vi "UHR-Fleezers Control (host) - 12.1.vi"() -> ()   [LabVIEW 2012] (continued)
            n2501 = xnode "Read/Write Control"("FPGA VI Reference In"=w4155, "error in"=w4154, "Green Filter Flipper"=FALSE) -> ("error out"=w4153:errorcluster)  [unwired: 1 out]
          }
        }
      }
      event "Pump 1 contents", "Pump 3 contents": Value Change {
        n2502 = event-data() -> ()  [unwired: 7 out]
        n2503 = local read "Pump 1 contents"() -> (→"Pump 1 cont disp":string)
        n2504 = local read "Pump 3 contents"() -> (→"Pump 3 cont disp":string)
      }
      event "Reset Trap Pos. FB": Value Change {
        n2505 = event-data() -> ()  [unwired: 7 out]
        n2506 = xnode "Read/Write Control"("FPGA VI Reference In"=w4161, "error in"=w4160, "Trap Pos. FB Reset"="Reset Trap Pos. FB") -> ()  [unwired: 2 out]
      }
      event "Rem fb disp offset": Value Change {
        n2507 = event-data() -> ()  [unwired: 7 out]
        n2508 = local write "Rem fb disp offset"(FALSE ("Rem fb disp offset")) -> ()
        n2509 = local read "Mean T1 Position (nm)"() -> (w4163:dbl)
        n2510 = local read "FB Trap Pos Offset"() -> (w4164:dbl)
        n2511 = Subtract(x=w4164, y=w4163) -> (x-y=w4162:dbl)
        n2512 = local write "FB Trap Pos Offset"(w4162) -> ()
      }
      event "Threshold (nm)": Value Change {
        n2513 = event-data() -> ()  [unwired: 7 out]
        n2514 = flat-sequence {
          tunnel: w4168 -> [w4176]
          tunnel: w4167 -> [w4175]
          tunnel: [w4169] -> w4166
          tunnel: w4166 -> [w4182]
          frame #0 {
            n2515 = xnode "Read/Write Control"("FPGA VI Reference In"=w4176, "error in"=w4175) -> ("FPGA VI Reference Out"=w4172:T18, "error out"=w4171:errorcluster, "FPGA TTrig Thresh"=w4173:i64)
            n2516 = local read "Threshold stored (nm)"() -> (w4181:dbl)
            n2517 = local read "Threshold (nm)"() -> (w4169:dbl)
            n2518 = local read "AOM X Cal (nm/MHz)"() -> (w4179:dbl)
            n2519 = Subtract(x=w4169, y=w4181) -> (x-y=w4180:dbl)
            n2520 = Divide(x=w4180, y=w4179) -> (x/y=w4177:dbl)
            n2521 = call "IR AOM freq to word.vi"("Frequency In (MHz)"=w4177) -> ("Frequency Word Out (double)"=w4178:dbl)
            n2522 = To Quad Integer(1:w4178) -> (0:w4174:i64)
            n2523 = Add(x=w4173, y=w4174) -> (x+y=w4170:i64)
            n2524 = xnode "Read/Write Control"("FPGA VI Reference In"=w4172, "error in"=w4171, "FPGA TTrig Thresh"=w4170) -> ()  [unwired: 2 out]
          }
          frame #1 {
            "Threshold stored (nm)" <- w4182
          }
        }
      }
      event "FB Trig Integrate": Value Change {
        n2525 = event-data() -> ()  [unwired: 7 out]
        n2526 = local read "FB Trig Integrate"() -> (w4184:u32)
        n2527 = xnode "Read/Write Control"("FPGA VI Reference In"=w4186, "error in"=w4185, "FB Trig Integrate"=w4184) -> ("error out"=w4183:errorcluster)  [unwired: 1 out]
      }
      event "11": Value Change {
        n2528 = event-data() -> ()  [unwired: 7 out]
        n2529 = local read "11"() -> (w4187:bool)
        n2530 = case shown="True" w4187 {
          frame False {
          }
          frame True {
            n2531 = local read "Messages"() -> (w4189:string)
            n2532 = call "Update messages.vi"("Message to add"="You kicked it up to 11!", "Old message string"=w4189) -> ("New message string"=w4190:string)
            n2533 = call <vilib>:"Beep.vi"() -> ()  [unwired: 12 in]
            n2534 = local write "Messages"(w4190) -> ()
          }
        }
      }
      event "Trap Pos. FB ON": Value Change {
        n2535 = event-data() -> ()  [unwired: 7 out]
        n2536 = xnode "Read/Write Control"("FPGA VI Reference In"=w4193, "error in"=w4192, "Force feedback"="Trap Pos. FB ON") -> ()  [unwired: 2 out]
      }
      event "Remove Action Offset": Value Change {
        n2537 = event-data() -> ()  [unwired: 7 out]
        n2538 = local write "Remove Action Offset"(FALSE ("Remove Action Offset")) -> ()
        n2539 = local read "Trap Pos. FB Mult Factor"() -> (w4198:i64)
        n2540 = local read "Trap Pos FB Action"() -> (w4196:i64)
        n2541 = local read "Trap Pos. FB Offset Factor"() -> (w4194:i64)
        n2542 = Multiply(x=w4198, y=w4196) -> (x*y=w4197:i64)
        n2543 = Add(x=w4197, y=w4194) -> (x+y=w4195:i64)
        n2544 = local write "Trap Pos. FB Offset Factor"(w4195) -> ()
        n2545 = xnode "Read/Write Control"("FPGA VI Reference In"=w4201, "error in"=w4200, "Trap Pos. FB Offset Factor"=w4195) -> ()  [unwired: 2 out]
      }
      event "Remove Unwinding Offset": Value Change {
        n2546 = event-data() -> ()  [unwired: 7 out]
        n2547 = local write "Remove Unwinding Offset"(FALSE ("Remove Action Offset")) -> ()
        n2548 = local read "Trap Pos. FB Mult Factor"() -> (w4213:i64)
        n2549 = local read "Trap Pos FB Action"() -> (w4211:i64)
        n2550 = local read "Trap Pos. FB Offset Factor"() -> (w4210:i64)
        n2551 = Multiply(x=w4213, y=w4211) -> (x*y=w4212:i64)
        n2552 = local read "Trap Pos. FB Mult Factor"() -> (w4209:i64)
        n2553 = Add(x=w4212, y=w4210) -> (x+y=w4203:i64)
        n2554 = Multiply(x=32768, y="factor") -> (x*y=w4206:dbl)
        n2555 = Multiply(x=w4206, y=w4209) -> (x*y=w4208:dbl)
        n2556 = Subtract(x=w4203, y=w4208) -> (x-y=w4207:dbl)
        n2557 = To Quad Integer(1:w4207) -> (0:w4202:i64)
        n2558 = xnode "Read/Write Control"("FPGA VI Reference In"=w4216, "error in"=w4215, "Trap Pos. FB Offset Factor"=w4202) -> ()  [unwired: 2 out]
        n2559 = local write "Trap Pos. FB Offset Factor"(w4202) -> ()
      }
      event "Trap Pos. FB Range", "Trap Pos. FB Gains", "Trap Pos. FB Mult Factor", "Trap Pos. FB Offset Factor", "Trap Pos FB Negate Action", "Trap Pos FB Monitor\nT1 or T2", "Differential FB?", "Negate Diff?": Value Change {
        n2560 = event-data() -> ()  [unwired: 7 out]
        n2561 = Unbundle By Name("Trap Pos. FB Gains") -> ("proportional gain (Kc)"=w4219:fxp<+/-,16,8>, "integral gain (Kc*Ts/Ti)"=w4218:fxp<+/-,16,8>, "derivative gain (Kc*Td/Ts)"=w4217:fxp<+/-,16,8>)
        n2562 = local read "Negate Diff?"() -> (w4224:bool)
        n2563 = Unbundle By Name("Trap Pos. FB Range") -> ("output high"=w4222:fxp<+/-,16,1>, "output low"=w4221:fxp<+/-,16,1>)
        n2564 = xnode "Read/Write Control"("FPGA VI Reference In"=w4232, "error in"=w4231, "FB2 output high"=w4222, "FB2 output low"=w4221, "P2"=w4219, "I2"=w4218, "D2"=w4217, "Trap Pos. FB Mult Factor"="Trap Pos. FB Mult Factor", "Trap Pos. FB Offset Factor"="Trap Pos. FB Offset Factor", "Trap Pos FB Negate Action"="Trap Pos FB Negate Action", "Trap Pos FB Monitor T1 or T2"="Trap Pos FB Monitor\nT1 or T2", "AI1 X Scale"="Trap Pos. AI1 X Pre-scale", "Negate Diff?"=w4224, "Diff FB Measurement?"="Differential FB?") -> ()  [unwired: 2 out]
      }
      event "Trap Pos FB SP", "Trap Pos FB SP 2", "Use SP 2": Value Change {
        n2565 = event-data() -> ()  [unwired: 7 out]
        n2566 = Select(t="Trap Pos FB SP 2", s="Use SP 2", f="Trap Pos FB SP") -> (s? t:f=w4233:fxp<+/-,16,1>)
        n2567 = xnode "Read/Write Control"("FPGA VI Reference In"=w4238, "error in"=w4237, "Trap Pos. FB SP"=w4233) -> ()  [unwired: 2 out]
      }
      event "Offset SP2 from SP1": Value Change {
        n2568 = event-data() -> ()  [unwired: 7 out]
        n2569 = local read "Trap Pos FB SP"() -> (w4241:fxp<+/-,16,1>)
        n2570 = Add(x=w4241, y="SP2 Offset") -> (x+y=w4239:fxp<+/-,16,1>)
        n2571 = property on="Trap Pos FB SP 2" class="DigNum (strict)"("Val(Sgnl)"=w4239) -> ()  [unwired: 2 in, 2 out]
        n2572 = local write "Offset SP2 from SP1"(FALSE ("Offset SP2 from SP1")) -> ()
      }
      event "Set Reading to\nSetpoint": Value Change {
        # "This is the actual PID input signal"
        n2573 = event-data() -> ()  [unwired: 7 out]
        n2574 = local write "Set Reading to\nSetpoint"(FALSE ("Set SP to Reading")) -> ()
        n2575 = xnode "Read/Write Control"("FPGA VI Reference In"=w4247, "error in"=w4246) -> ("FPGA VI Reference Out"=w4245:T18, "error out"=w4244:errorcluster, "Trap Pos FB Int-Norm Signal"=w4243:fxp<+/-,16,1>)
        n2576 = local read "Differential FB?"() -> (w4248:bool)
        n2577 = case shown="False" w4248 {
          tunnel: [w4253 w4260] -> w4250
          tunnel: w4243 -> [w4251 w4260]
          frame False {
            n2578 = local read "Trap Pos FB Monitor\nT1 or T2"() -> (w4256:bool)
            n2579 = local read "Trap X AI1 (DMA)"() -> (w4259:T13)
            n2580 = Unbundle By Name(w4259) -> ("Set 1"=w4258:fxp<+/-,16,1>, "Set 2"=w4257:fxp<+/-,16,1>)
            n2581 = Select(t=w4258, s=w4256, f=w4257) -> (s? t:f=w4255:fxp<+/-,16,1>)
            n2582 = Not(x="Set SP Using...") -> (.not. x?=w4252:bool)
            n2583 = Select(t=w4251, s=w4252, f=w4255) -> (s? t:f=w4253:fxp<+/-,16,1>)
          }
          frame True {
          }
        }
        n2584 = xnode "Read/Write Control"("FPGA VI Reference In"=w4245, "error in"=w4244, "Trap Pos. FB SP"=w4250) -> ()  [unwired: 2 out]
        n2585 = local write "Trap Pos FB SP"(w4250) -> ()
      }
      event "Trap Pos. FB Out Scale 2^n": Value Change {
        n2586 = event-data() -> ()  [unwired: 7 out]
        n2587 = Scale By Power Of 2(n="Trap Pos. FB Out Scale 2^n", x=ext 1.0) -> (x*2^n=w4261:ext)
        n2588 = property on="Trap Pos. FB Mult Factor" class="DigNum (strict)"("Val(Sgnl)"=w4261) -> ()  [unwired: 2 in, 2 out]
      }
      event "Trap Pos FB Int Count": Value Change {
        n2589 = event-data() -> ()  [unwired: 7 out]
        n2590 = xnode "Read/Write Control"("FPGA VI Reference In"=w4266, "error in"=w4265, "Trap Pos FB Int Count"="Trap Pos FB Int Count") -> ()  [unwired: 2 out]
      }
      event "Trap pos": Value Change {
        n2591 = event-data() -> ()  [unwired: 7 out]
        n2592 = case shown="True" "Trap pos" {
          frame False {
            n2593 = property on="Trap Delta Graph" class="WFGraph (strict)"("Visible"=TRUE) -> ()  [unwired: 2 in, 2 out]
            n2594 = property on="Saved trap pos" class="WFGraph (strict)"("Visible"=FALSE) -> ()  [unwired: 2 in, 2 out]
          }
          frame True {
            n2595 = property on="Saved trap pos" class="WFGraph (strict)"("Visible"=TRUE) -> ()  [unwired: 2 in, 2 out]
            n2596 = property on="Trap Delta Graph" class="WFGraph (strict)"("Visible"=FALSE) -> ()  [unwired: 2 in, 2 out]
          }
        }
      }
    }
    "error out 2" <- w3161
    n2597 = node-c288() -> ()  [unwired: 2 out]
  }
  n2598 = timed-loop "Oscillate Trap/AOM (fishing, debugging)" {
    tunnel: w28 -> [w4273]
    tunnel: [w4272] -> w119
    timing: w114 -> [_]
    timing-out: [_] -> w113
    stop <- w4272 stop-if-true
    n2599 = node-c288() -> ()  [unwired: 2 out]
    n2600 = event shown="[0] \"Oscillate Set 1\", \"Fish for Tether\": Value Change" {
      selector: _ -> [_ _ _]
      dyn-events: _ -> [_ _ _]
      timeout: _ -> [_ _ _]
      tunnel: w4273 -> [w4280 _ _]
      tunnel: [FALSE ("Stop All") _ w4869] -> w4272
      event "Oscillate Set 1", "Fish for Tether": Value Change {
        n2601 = event-data() -> ()  [unwired: 6 out]
        n2602 = local read "Oscillate Set 1"() -> (w4279:bool)
        n2603 = Or(x=w4279, y="Fish for Tether") -> (x .or. y?=w4277:bool)
        n2604 = case shown="True" w4277 {
          tunnel: w4280 -> [_ w4283]
          tunnel: "Fish for Tether" -> [_ w4282]
          frame False {
          }
          frame True {
            n2605 = case shown="True" w4282 {
              selector: w4282 -> [w4286 w4292]
              tunnel: [w4286 w4292] -> w4281
              frame False {
              }
              frame True {
                n2606 = local write "Scan axis 2"(TRUE) -> ()
                n2607 = local write "Tether"(FALSE ("Tether")) -> ()
                n2608 = local read "Flow ON during cal?"() -> (w4287:bool)
                n2609 = property on="Trap Delta (MHz)" class="DigNum (strict)"("Val(Sgnl)"="Furthest Delta (MHz)") -> ()  [unwired: 2 in, 2 out]
                n2610 = Or(x="Flow ON during \nfishing?", y=w4287) -> (x .or. y?=w4288:bool)
                n2611 = Wait (ms)(milliseconds to wait=u32 500) -> ()  [unwired: 1 out]
                n2612 = property on="Sample Channel\nFlow" class="Bool (strict)"("Val(Sgnl)"=w4288) -> ()  [unwired: 2 in, 2 out]
              }
            }
            n2613 = node-c288() -> (w4285:T20)  [unwired: 4 out]
            n2614 = timed-loop "Oscillate AOD" {
              timing: w4285 -> [_]
              timing-out: [_] -> w4284
              tunnel: w4283 -> [w4302]
              tunnel: w4281 -> [w4295]
              i -> [w4304]
              stop <- w4301 stop-if-true
              n2615 = node-c288() -> (w4303:i64)  [unwired: 1 out]
              n2616 = flat-sequence {
                tunnel: w4304 -> [w4331]
                tunnel: w4303 -> [w4330]
                tunnel: w4302 -> [w4309]
                tunnel: w4295 -> [w4312]
                tunnel: [w4312] -> w4300
                tunnel: [w4311] -> w4299
                tunnel: [w4308] -> w4298
                tunnel: [w4305] -> w4296
                tunnel: w4300 -> [w4367]
                tunnel: w4299 -> [w4365]
                tunnel: w4298 -> [w4364]
                tunnel: [w4363] -> w4297
                tunnel: w4296 -> [w4362]
                tunnel: [w4439] -> w4301
                tunnel: w4297 -> [w4438]
                frame #0 {
                  n2617 = Divide(x=w4330, y=i64 1000) -> (x/y=w4325:dbl)
                  n2618 = Multiply(x=w4325, y=w4331) -> (x*y=w4327:dbl)
                  n2619 = local read "BD 1 Frequency 2 (MHz)"() -> (w4310:dbl)
                  n2620 = Multiply(x="Osc. freq. (Hz)", y=6.283185307179586) -> (x*y=w4328:dbl)
                  n2621 = Multiply(x=w4328, y=w4327) -> (x*y=w4307:dbl)
                  n2622 = local read "BD 1 Frequency 1 (MHz)"() -> (w4315:dbl)
                  n2623 = local read "BD 2 Frequency 1 (MHz)"() -> (w4314:dbl)
                  n2624 = case shown="True" w4312 {
                    tunnel: w4307 -> [w4337 w4342]
                    tunnel: w4315 -> [_ w4353]
                    tunnel: w4310 -> [_ w4354]
                    tunnel: [w4334 w4348] -> w4313
                    tunnel: [FALSE w4345] -> w4308
                    tunnel: [0.0 w4338] -> w4305
                    frame False {
                      n2625 = Sine(x=w4337) -> (sin(x)=w4335:dbl)
                      n2626 = Multiply(x=w4335, y="Osc. amp. (MHz)") -> (x*y=w4334:dbl)
                    }
                    frame True {
                      n2627 = Cosine(x=w4342) -> (cos(x)=w4357:dbl)
                      n2628 = Subtract(x=w4354, y=w4353) -> (x-y=w4352:dbl)
                      n2629 = Decrement(x=w4357) -> (x-1=w4356:dbl)
                      n2630 = Subtract(x=w4352, y="Closest Delta (MHz)") -> (x-y=w4349:dbl)
                      n2631 = Divide(x=w4356, y=-2.0) -> (x/y=w4350:dbl)
                      n2632 = Multiply(x=w4350, y=w4349) -> (x*y=w4348:dbl)
                      n2633 = local read "Vec Mean of T1 T2"() -> (w4344:dbl[])
                      n2634 = Greater?(x=w4344, y="Stop F (pN)") -> (0:w4346:bool[])
                      n2635 = Or Array Elements(Boolean array=w4346) -> (logical OR=w4345:bool)
                      n2636 = Divide(x=w4342, y=6.283185307179586) -> (x/y=w4341:dbl)
                      n2637 = Round Toward +Infinity(x=w4341) -> (ceil(x): smallest int >= x=w4338:dbl)
                      "Attempts" <- w4338
                      n2638 = Greater?(x=w4338, y="Attempt Limit") -> (0:w4340:bool)
                      n2639 = case shown="True" w4340 {
                        frame False {
                        }
                        frame True {
                          n2640 = local write "Fish for Tether"(FALSE ("Fish for Tether")) -> ()
                          n2641 = call <vilib>:"Beep.vi"() -> ()  [unwired: 3 in, 9 out]
                          n2642 = local read "Messages"() -> (w4359:string)
                          n2643 = call "Update messages.vi"("Message to add"="Tether fishing timeout." ("Messages"), "Old message string"=w4359) -> ("New message string"=→"Messages":string)
                        }
                      }
                    }
                  }
                  n2644 = Select(t=w4315, s="Scan axis 2", f=w4314) -> (s? t:f=w4318:dbl)
                  n2645 = Add(x=w4313, y=w4318) -> (x+y=w4311:dbl)
                  n2646 = Select(t=w4311, s="Scan axis 2", f=w4315) -> (s? t:f=w4321:dbl)
                  n2647 = Select(t=w4314, s="Scan axis 2", f=w4311) -> (s? t:f=w4320:dbl)
                  n2648 = local read "Y RF Frequency Limits (MHz)"() -> (w4316:T15)
                  n2649 = local read "X RF Frequency Limits (MHz)"() -> (w4317:T15)
                  n2650 = local read "BD 1 Frequency 3 (MHz)"() -> (w4324:dbl)
                  n2651 = local read "BD 2 Frequency 2 (MHz)"() -> (w4323:dbl)
                  n2652 = local read "BD 2 Frequency 3 (MHz)"() -> (w4322:dbl)
                  n2653 = call "set RF board frequency - interlace.vi"("Board 2 Frequency Limits"=w4316, "Board 1 Frequency Limits"=w4317, "FPGA VI Reference In"=w4309, "Board 2 Frequency 3 (MHz)"=w4322, "Board 1 Frequency 3 (MHz)"=w4324, "Board 2 Frequency 2 (MHz)"=w4323, "Board 2 Frequency 1 (MHz)"=w4320, "Board 1 Frequency 2 (MHz)"=w4310, "Board 1 Frequency 1  (MHz)"=w4321) -> ()  [unwired: 1 in, 2 out]
                }
                frame #1 {
                  n2654 = And(x=w4367, y=w4364) -> (x .and. y?=w4366:bool)
                  n2655 = case "Only if were fishing and now formed tether" shown="False" w4366 {
                    tunnel: w4365 -> [w4369 w4384]
                    tunnel: [w4368 w4383] -> w4363
                    tunnel: w4362 -> [_ w4379]
                    frame False {
                      n2656 = local read "Fish for Tether"() -> (w4368:bool)
                      n2657 = case shown="False" w4368 {
                        tunnel: w4369 -> [w4370 _]
                        frame False {
                          n2658 = property on="BD 1 Frequency 1 (MHz)" class="DigNum (strict)"("Val(Sgnl)"=w4370) -> ()  [unwired: 2 in, 2 out]
                        }
                        frame True {
                        }
                      }
                    }
                    frame True {
                      w4383 = FALSE ("Fish for Tether")
                      n2659 = call <vilib>:"Beep.vi"() -> ()  [unwired: 3 in, 9 out]
                      n2660 = Number To Decimal String(number=w4379, width (-)=i16 1) -> (decimal integer string=w4377:string)
                      n2661 = Concatenate Strings("Formed tether in ", w4377, " attempt(s)." ("string")) -> (w4374:string)
                      n2662 = local read "Messages"() -> (w4381:string)
                      n2663 = local write "Fish for Tether"(w4383) -> ()
                      n2664 = call "Update messages.vi"("Message to add"=w4374, "Old message string"=w4381) -> ("New message string"=w4380:string)
                      n2665 = local write "Messages"(w4380) -> ()
                      n2666 = Get Date/Time In Seconds() -> (seconds since 1Jan1904=→"Time tether formed":timestamp)
                      n2667 = local read "Flow ON during cal?"() -> (w4371:bool)
                      n2668 = property on="Sample Channel\nFlow" class="Bool (strict)"("Val(Sgnl)"=w4371) -> (error out=w4372:errorcluster)  [unwired: 2 in, 1 out]
                      n2669 = case shown="\"2\", \"3\", \"4\", \"5\", \"6\"" "Then..." {
                        selector: "Then..." -> [_ w4387]
                        tunnel: w4384 -> [w4386 _]
                        tunnel: w4372 -> [_ _]
                        frame "1", Default {
                          n2670 = property on="BD 1 Frequency 1 (MHz)" class="DigNum (strict)"("Val(Sgnl)"=w4386) -> ()  [unwired: 2 in, 2 out]
                        }
                        frame "2", "3", "4", "5", "6" {
                          n2671 = flat-sequence {
                            tunnel: w4387 -> [w4389]
                            frame #0 {
                              n2672 = property on="Trap Delta (MHz)" class="DigNum (strict)"("Val(Sgnl)"="Move to Delta 1 (MHz)") -> ()  [unwired: 2 in, 2 out]
                            }
                            frame #1 {
                              n2673 = case shown="\"5\", \"6\"" w4389 {
                                selector: w4389 -> [w4392 w4402 _]
                                frame "3", "4" {
                                n2674 = flat-sequence {
                                tunnel: w4392 -> [w4393]
                                tunnel: [w4393] -> w4390
                                tunnel: [w4395] -> w4391
                                tunnel: w4390 -> [w4395]
                                tunnel: w4391 -> [w4399]
                                frame #0 {
                                n2675 = property on="Green Laser ON/Interlacing" class="Bool (strict)"("Val(Sgnl)"=TRUE ("Value (Signaling)")) -> ()  [unwired: 2 in, 2 out]
                                }
                                frame #1 {
                                n2676 = Multiply(x="Wait Before Save (s)", y=u32 1000 ("x")) -> (x*y=w4397:u32)
                                n2677 = Wait (ms)(milliseconds to wait=w4397) -> ()  [unwired: 1 out]
                                }
                                frame #2 {
                                n2678 = property on="Start Saving" class="Bool (strict)"("Value"=TRUE ("Start Saving")) -> ()  [unwired: 2 in, 2 out]
                                n2679 = case shown="\"4\"" w4399 {
                                frame Default {
                                }
                                frame "4" {
                                n2680 = property on="Fl. Triggered..." class="Bool (strict)"("Val(Sgnl)"=TRUE ("Value (Signaling)")) -> ()  [unwired: 2 in, 2 out]
                                }
                                }
                                }
                                }
                                }
                                frame "5", "6" {
                                n2681 = stacked-sequence {
                                tunnel: w4402 -> [_ _ _ _ _ _ w4414]
                                frame #0 {
                                n2682 = Replace Array Subset(array=u32[] [0] ("Index Values"), new element="Raster Set Upon Tether", index=0) -> (w4403:u32[])
                                n2683 = property on="Saved AOD Raster Scan Parameter Sets" class="Arr (strict)"("Index Values"=w4403) -> ()  [unwired: 2 in, 2 out]
                                }
                                frame #1 {
                                n2684 = Wait (ms)(milliseconds to wait=u32 500) -> ()  [unwired: 1 out]
                                }
                                frame #2 {
                                n2685 = property on="Load parameters" class="Bool (strict)"("Val(Sgnl)"=TRUE ("Value (Signaling)")) -> ()  [unwired: 2 in, 2 out]
                                n2686 = case shown="True" "Green ON During Raster" {
                                frame False {
                                }
                                frame True {
                                n2687 = property on="Green Laser ON/Interlacing" class="Bool (strict)"("Val(Sgnl)"=TRUE ("Value (Signaling)")) -> ()  [unwired: 2 in, 2 out]
                                }
                                }
                                }
                                frame #3 {
                                n2688 = Wait (ms)(milliseconds to wait=u32 500) -> ()  [unwired: 1 out]
                                }
                                frame #4 {
                                n2689 = property on="Trap Raster Scan" class="Bool (strict)"("Val(Sgnl)"=TRUE ("Value (Signaling)")) -> ()  [unwired: 2 in, 2 out]
                                }
                                frame #5 {
                                n2690 = Wait (ms)(milliseconds to wait=u32 2000) -> ()  [unwired: 1 out]
                                }
                                frame #6 {
                                n2691 = flat-sequence {
                                tunnel: w4414 -> [w4421]
                                frame #0 {
                                n2692 = while {
                                stop <- w4417 stop-if-true
                                n2693 = local read "Raster Scanning..."() -> (w4416:bool)
                                n2694 = local read "Saving..."() -> (w4419:bool)
                                n2695 = Wait (ms)(milliseconds to wait=u32 100) -> ()  [unwired: 1 out]
                                n2696 = Not(x=w4419) -> (.not. x?=w4418:bool)
                                n2697 = Not(x=w4416) -> (.not. x?=w4415:bool)
                                n2698 = And(x=w4418, y=w4415) -> (x .and. y?=w4417:bool)
                                }
                                }
                                frame #1 {
                                n2699 = local read "Tether"() -> (w4422:bool)
                                n2700 = case shown="True" w4422 {
                                tunnel: w4421 -> [_ w4424]
                                frame False {
                                n2701 = property on="Fish for Tether" class="Bool (strict)"("Val(Sgnl)"="Fish again after \nraster break?") -> ()  [unwired: 2 in, 2 out]
                                }
                                frame True {
                                n2702 = stacked-sequence {
                                tunnel: w4424 -> [_ w4428 _ _]
                                frame #0 {
                                n2703 = property on="Trap Delta (MHz)" class="DigNum (strict)"("Val(Sgnl)"="Move to Delta 2 (MHz)") -> ()  [unwired: 2 in, 2 out]
                                n2704 = case shown="True" "Flow ON after\ntether testing?" {
                                frame False {
                                }
                                frame True {
                                n2705 = property on="Sample Channel\nFlow" class="Bool (strict)"("Val(Sgnl)"=TRUE ("Value (Signaling)")) -> ()  [unwired: 2 in, 2 out]
                                }
                                }
                                }
                                frame #1 {
                                n2706 = flat-sequence {
                                tunnel: w4428 -> [w4430]
                                frame #0 {
                                n2707 = Wait (ms)(milliseconds to wait=u32 500) -> ()  [unwired: 1 out]
                                }
                                frame #1 {
                                n2708 = case shown="\"6\"" w4430 {
                                frame Default {
                                }
                                frame "6" {
                                n2709 = property on="Green Laser ON/Interlacing" class="Bool (strict)"("Val(Sgnl)"=TRUE ("Green Laser ON/Interlacing")) -> ()  [unwired: 2 in, 2 out]
                                }
                                }
                                }
                                frame #2 {
                                n2710 = Wait (ms)(milliseconds to wait=u32 500) -> ()  [unwired: 1 out]
                                }
                                frame #3 {
                                n2711 = local write "Start Saving"("Save at end (5, 6)") -> ()
                                }
                                }
                                }
                                frame #2 {
                                n2712 = local read "Bead Sep. Int. Time (s)"() -> (w4436:dbl)
                                n2713 = Multiply(x=w4436, y=1000.0) -> (x*y=w4435:dbl)
                                n2714 = Wait (ms)(milliseconds to wait=w4435) -> ()  [unwired: 1 out]
                                }
                                frame #3 {
                                n2715 = property on="Remove Offset" class="Bool (strict)"("Val(Sgnl)"=TRUE ("Value (Signaling)")) -> ()  [unwired: 2 in, 2 out]
                                }
                                }
                                }
                                }
                                }
                                }
                                }
                                }
                                }
                                frame "2", Default {
                                }
                              }
                            }
                          }
                        }
                      }
                      "Tether" <- "Tether Alarm?"
                    }
                  }
                }
                frame #2 {
                  n2716 = local read "Oscillate Set 1"() -> (w4443:bool)
                  n2717 = local read "Stop All"() -> (w4441:bool)
                  n2718 = Or(x=w4443, y=w4438) -> (x .or. y?=w4440:bool)
                  n2719 = Not(x=w4440) -> (.not. x?=w4442:bool)
                  n2720 = Compound Arithmetic op=OR(w4441, w4442) -> (w4439:bool)
                }
              }
              n2721 = node-c288() -> ()  [unwired: 2 out]
            }
            n2722 = node-c288(w4284) -> ()  [unwired: 1 out]
          }
        }
      }
      event "Fl. Triggered...": Value Change {
        n2723 = event-data() -> ()  [unwired: 7 out]
        n2724 = case shown="True" "Fl. Triggered..." {
          frame False {
          }
          frame True {
            n2725 = node-c288() -> (w4454:T20)  [unwired: 4 out]
            n2726 = timed-loop {
              timing: w4454 -> [_]
              timing-out: [_] -> w4453
              tunnel: "Action" -> [w4462]
              shift-right: [w4459] -> _
              shift-left: u8 255 -> [w4461]
              shift-right: [w4456] -> _
              shift-left: 255 -> [w4458]
              stop <- w4455 stop-if-true
              # "Reset confocal spot"
              n2727 = node-c288() -> ()  [unwired: 2 out]
              n2728 = flat-sequence {
                tunnel: w4462 -> [w4482]
                tunnel: w4461 -> [w4481]
                tunnel: [w4480] -> w4460
                tunnel: w4458 -> [w4467]
                tunnel: [w4466] -> w4457
                tunnel: [w4861] -> w4455
                tunnel: w4460 -> [w4860]
                tunnel: [w4860] -> w4459
                tunnel: [w4859] -> w4456
                tunnel: w4457 -> [w4859]
                frame #0 {
                  n2729 = local read "Delta Fl. 2"() -> (w4479:dbl)
                  n2730 = local read "Delta Fl. 1"() -> (w4474:dbl)
                  n2731 = Multiply(x="Fl. Delta Thresh. (kHz)", y=1000.0) -> (x*y=w4469:dbl)
                  n2732 = Select(t=w4474, s="APD to Watch", f=w4479) -> (s? t:f=w4470:dbl)
                  n2733 = Greater?(x=w4470, y=w4469) -> (0:w4475:bool)
                  n2734 = Or(x="Force Yank", y=w4475) -> (x .or. y?=w4473:bool)
                  n2735 = And(x=w4473, y="Yank when?") -> (x .and. y?=w4471:bool)
                  n2736 = case shown="False" w4471 {
                    tunnel: w4482 -> [w4485 w4686]
                    tunnel: w4481 -> [w4487 w4682]
                    tunnel: [w4487 w4680] -> w4480
                    tunnel: w4470 -> [w4493 _]
                    tunnel: w4469 -> [w4492 _]
                    tunnel: "Force Yank" -> [w4490 _]
                    tunnel: w4467 -> [w4489 w4679]
                    tunnel: [w4488 w4679] -> w4466
                    frame False {
                      n2737 = Negate(x=w4492) -> (-x=w4484:dbl)
                      n2738 = local write "Fl. High"(TRUE ("Fl. High")) -> ()
                      n2739 = Less?(x=w4493, y=w4484) -> (x < y?=w4491:bool)
                      n2740 = Or(x=w4490, y=w4491) -> (x .or. y?=w4486:bool)
                      n2741 = case shown="True" w4486 {
                        tunnel: w4489 -> [w4494 w4504]
                        tunnel: [w4494 w4503] -> w4488
                        tunnel: w4485 -> [_ w4502]
                        frame False {
                        }
                        frame True {
                          n2742 = flat-sequence {
                            tunnel: w4504 -> [w4510]
                            tunnel: w4502 -> [w4507]
                            tunnel: [w4509] -> w4501
                            tunnel: [w4508] -> w4500
                            tunnel: [w4507] -> w4499
                            tunnel: w4498 -> [w4506]
                            tunnel: [w4506] -> w4497
                            tunnel: w4496 -> [w4505]
                            tunnel: [w4505] -> w4495
                            tunnel: [w4581] -> w4503
                            tunnel: w4501 -> [w4581]
                            tunnel: w4500 -> [w4580]
                            tunnel: w4499 -> [w4579]
                            tunnel: w4497 -> [w4578]
                            tunnel: w4495 -> [w4577]
                            frame #0 {
                              n2743 = call <vilib>:"Beep.vi"() -> ()  [unwired: 12 in]
                              n2744 = local write "Waiting"(FALSE ("Waiting")) -> ()
                              n2745 = Increment(x=w4510) -> (x+1=w4509:i32)
                              n2746 = case shown="\"Yank\"" w4507 {
                                tunnel: w4509 -> [_ w4515 _]
                                frame "Alarm", Default {
                                }
                                frame "Yank" {
                                n2747 = flat-sequence {
                                tunnel: w4515 -> [w4518]
                                tunnel: [w4517] -> w4514
                                tunnel: [w4516] -> w4513
                                tunnel: w4514 -> [w4528]
                                tunnel: w4513 -> [w4529]
                                frame #0 {
                                n2748 = local read "Yank Delay (s)"() -> (w4521:dbl)
                                n2749 = local read "N Array El"() -> (w4516:u8)
                                n2750 = Quotient & Remainder(x=w4518, y=w4516) -> (x-y*floor(x/y)=w4517:i32)  [unwired: 1 out]
                                n2751 = Multiply(x=w4521, y=1000.0) -> (x*y=w4519:dbl)
                                n2752 = Wait (ms)(milliseconds to wait=w4519) -> ()  [unwired: 1 out]
                                }
                                frame #1 {
                                n2753 = local read "Yank to which?"() -> (w4523:bool)
                                n2754 = local read "Random Choice"() -> (w4533:bool)
                                n2755 = local read "Yank to Trap Delta (MHz)"() -> (w4526:dbl[])
                                n2756 = local read "Yank to SP"() -> (w4527:dbl[])
                                n2757 = Random Number (0-1)() -> (number: 0 to 1=w4532:dbl)
                                n2758 = Multiply(x=w4529, y=w4532) -> (x*y=w4531:dbl)
                                n2759 = Round Toward -Infinity(1:w4531) -> (0:w4530:dbl)
                                n2760 = Select(t=w4530, s=w4533, f=w4528) -> (s? t:f=w4524:dbl)
                                n2761 = Select(t=w4526, s=w4523, f=w4527) -> (s? t:f=w4525:dbl[])
                                n2762 = Index Array(array=w4525, index=w4524) -> (element=w4522:dbl)
                                n2763 = case shown="True" w4523 {
                                tunnel: w4522 -> [w4534 w4561]
                                frame False {
                                n2764 = flat-sequence {
                                tunnel: w4534 -> [w4535]
                                frame #0 {
                                n2765 = property on="Trap Pos FB SP" class="DigNum (strict)"("Val(Sgnl)"=w4535) -> ()  [unwired: 2 in, 2 out]
                                }
                                frame #1 {
                                n2766 = Wait (ms)(milliseconds to wait=u32 700) -> ()  [unwired: 1 out]
                                }
                                frame #2 {
                                n2767 = local read "Action (%)"() -> (w4540:dbl)
                                n2768 = Absolute Value(x=w4540) -> (abs(x)=w4539:dbl)
                                n2769 = Greater?(x=w4539, y=70.0) -> (0:w4537:bool)
                                n2770 = property on="Remove Action Offset" class="Bool (strict)"("Val(Sgnl)"=w4537) -> ()  [unwired: 2 in, 2 out]
                                }
                                frame #3 {
                                n2771 = for {
                                N: 4 -> [_]
                                n2772 = flat-sequence {
                                frame #0 {
                                n2773 = Wait (ms)(milliseconds to wait=u32 500) -> ()  [unwired: 1 out]
                                }
                                frame #1 {
                                n2774 = local read "Action (%)"() -> (w4546:dbl)
                                n2775 = Absolute Value(x=w4546) -> (abs(x)=w4545:dbl)
                                n2776 = Greater?(x=w4545, y=70.0) -> (0:w4543:bool)
                                n2777 = property on="Remove Action Offset" class="Bool (strict)"("Val(Sgnl)"=w4543) -> ()  [unwired: 2 in, 2 out]
                                }
                                }
                                }
                                }
                                frame #4 {
                                n2778 = Wait (ms)(milliseconds to wait=u32 500) -> ()  [unwired: 1 out]
                                }
                                frame #5 {
                                n2779 = local read "Mean"() -> (w4554:dbl)
                                n2780 = Greater?(x=w4554, y=11.0) -> (0:w4548:bool)
                                n2781 = Not(x=w4548) -> (.not. x?=w4549:bool)
                                n2782 = And(x=w4549, y="Shift confocal") -> (x .and. y?=w4551:bool)
                                n2783 = And(x=w4548, y="Shift confocal") -> (x .and. y?=w4552:bool)
                                n2784 = case shown="True" w4552 {
                                frame False {
                                }
                                frame True {
                                n2785 = local read "Confocal Y 2 (V)"() -> (w4558:dbl)
                                n2786 = local read "Confocal X 2 (V)"() -> (w4557:dbl)
                                n2787 = property on="AO1" class="Slide (strict)"("Val(Sgnl)"=w4558) -> ()  [unwired: 2 in, 2 out]
                                n2788 = property on="AO2" class="Slide (strict)"("Val(Sgnl)"=w4557) -> ()  [unwired: 2 in, 2 out]
                                }
                                }
                                n2789 = case shown="True" w4551 {
                                frame False {
                                }
                                frame True {
                                n2790 = local read "Confocal Y 1 (V)"() -> (w4556:dbl)
                                n2791 = local read "Confocal X 1 (V)"() -> (w4555:dbl)
                                n2792 = property on="AO1" class="Slide (strict)"("Val(Sgnl)"=w4556) -> ()  [unwired: 2 in, 2 out]
                                n2793 = property on="AO2" class="Slide (strict)"("Val(Sgnl)"=w4555) -> ()  [unwired: 2 in, 2 out]
                                }
                                }
                                }
                                frame #6 {
                                n2794 = Wait (ms)(milliseconds to wait=u32 1500) -> ()  [unwired: 1 out]
                                }
                                frame #7 {
                                n2795 = property on="Rem fb disp offset" class="Bool (strict)"("Val(Sgnl)"=TRUE ("Value (Signaling)")) -> ()  [unwired: 2 in, 2 out]
                                }
                                }
                                }
                                frame True {
                                n2796 = flat-sequence {
                                tunnel: w4561 -> [w4562]
                                frame #0 {
                                n2797 = property on="Trap Delta (MHz)" class="DigNum (strict)"("Val(Sgnl)"=w4562) -> ()  [unwired: 2 in, 2 out]
                                }
                                frame #1 {
                                n2798 = Wait (ms)(milliseconds to wait=u32 500) -> ()  [unwired: 1 out]
                                }
                                frame #2 {
                                n2799 = local read "Shift confocal"() -> (w4568:bool)
                                n2800 = local read "Mean"() -> (w4570:dbl)
                                n2801 = Greater?(x=w4570, y=11.0) -> (0:w4567:bool)
                                n2802 = Not(x=w4567) -> (.not. x?=w4566:bool)
                                n2803 = And(x=w4566, y=w4568) -> (x .and. y?=w4564:bool)
                                n2804 = And(x=w4567, y=w4568) -> (x .and. y?=w4565:bool)
                                n2805 = case shown="True" w4565 {
                                frame False {
                                }
                                frame True {
                                n2806 = local read "Confocal Y 2 (V)"() -> (w4574:dbl)
                                n2807 = local read "Confocal X 2 (V)"() -> (w4573:dbl)
                                n2808 = property on="AO2" class="Slide (strict)"("Val(Sgnl)"=w4573) -> ()  [unwired: 2 in, 2 out]
                                n2809 = property on="AO1" class="Slide (strict)"("Val(Sgnl)"=w4574) -> ()  [unwired: 2 in, 2 out]
                                }
                                }
                                n2810 = case shown="True" w4564 {
                                frame False {
                                }
                                frame True {
                                n2811 = local read "Confocal X 1 (V)"() -> (w4571:dbl)
                                n2812 = local read "Confocal Y 1 (V)"() -> (w4572:dbl)
                                n2813 = property on="AO2" class="Slide (strict)"("Val(Sgnl)"=w4571) -> ()  [unwired: 2 in, 2 out]
                                n2814 = property on="AO1" class="Slide (strict)"("Val(Sgnl)"=w4572) -> ()  [unwired: 2 in, 2 out]
                                }
                                }
                                }
                                }
                                }
                                }
                                }
                                }
                                }
                                frame "Image" {
                                n2815 = property on="Confocal Image" class="Bool (strict)"("Val(Sgnl)"=TRUE ("Value (Signaling)")) -> ()  [unwired: 2 in, 2 out]
                                }
                              }
                              n2816 = local write "Fl. High"(FALSE ("Fl. High")) -> ()
                              n2817 = local read "Time (s)"() -> (w4508:dbl)
                            }
                            frame #1 {
                              n2818 = case shown="True" "Auto F Reset" {
                                tunnel: w4580 -> [_ w4585]
                                tunnel: w4579 -> [_ w4584]
                                tunnel: w4578 -> [_ w4583]
                                tunnel: w4577 -> [_ w4582]
                                frame False {
                                }
                                frame True {
                                n2819 = node-c288() -> (w4587:T20)  [unwired: 4 in]
                                n2820 = timed-loop {
                                timing: w4587 -> [_]
                                timing-out: [_] -> w4586
                                tunnel: w4585 -> [w4592]
                                tunnel: w4584 -> [w4591]
                                tunnel: w4583 -> [w4590]
                                tunnel: w4582 -> [w4589]
                                stop <- w4588 stop-if-true
                                n2821 = node-c288() -> ()  [unwired: 1 in, 1 out]
                                n2822 = local read "Fl. Delta Thresh. (kHz)"() -> (w4601:dbl)
                                n2823 = local read "APD to Watch"() -> (w4602:bool)
                                n2824 = local read "Delta Fl. 1"() -> (w4603:dbl)
                                n2825 = local read "Delta Fl. 2"() -> (w4604:dbl)
                                n2826 = local read "Fl. Triggered..."() -> (w4595:bool)
                                n2827 = local read "Stop All"() -> (w4596:bool)
                                n2828 = local read "Reset Force"() -> (w4594:bool)
                                n2829 = Multiply(x=w4601, y=1000.0) -> (x*y=w4599:dbl)
                                n2830 = Not(x=w4595) -> (.not. x?=w4593:bool)
                                n2831 = Select(t=w4603, s=w4602, f=w4604) -> (s? t:f=w4598:dbl)
                                n2832 = Greater?(x=w4598, y=w4599) -> (0:w4597:bool)
                                n2833 = Compound Arithmetic op=OR(w4597, w4596, w4593, w4594) -> (w4588:bool)
                                n2834 = case shown="True" w4588 {
                                tunnel: w4592 -> [_ w4608]
                                tunnel: w4591 -> [_ w4612]
                                tunnel: w4590 -> [_ w4611]
                                tunnel: w4589 -> [_ w4610]
                                frame False {
                                }
                                frame True {
                                n2835 = case shown="\"Yank\"" w4612 {
                                tunnel: w4611 -> [_ w4622]
                                tunnel: w4610 -> [_ w4620]
                                frame "Image", Default {
                                }
                                frame "Yank" {
                                n2836 = flat-sequence {
                                tunnel: [w4625] -> w4623
                                tunnel: w4622 -> [w4625]
                                tunnel: [w4624] -> w4621
                                tunnel: w4620 -> [w4624]
                                tunnel: w4623 -> [w4631]
                                tunnel: w4621 -> [w4629]
                                frame #0 {
                                n2837 = local read "Yank Delay (s)"() -> (w4628:dbl)
                                n2838 = Multiply(x=w4628, y=1000.0) -> (x*y=w4626:dbl)
                                n2839 = Wait (ms)(milliseconds to wait=w4626) -> ()  [unwired: 1 out]
                                }
                                frame #1 {
                                n2840 = local read "Yank to which?"() -> (w4630:bool)
                                n2841 = case shown="False" w4630 {
                                tunnel: w4631 -> [_ w4659]
                                tunnel: w4629 -> [w4632 _]
                                frame False {
                                n2842 = flat-sequence {
                                tunnel: w4632 -> [w4633]
                                frame #0 {
                                n2843 = property on="Trap Pos FB SP" class="DigNum (strict)"("Val(Sgnl)"=w4633) -> ()  [unwired: 2 in, 2 out]
                                }
                                frame #1 {
                                n2844 = Wait (ms)(milliseconds to wait=u32 700) -> ()  [unwired: 1 out]
                                }
                                frame #2 {
                                n2845 = local read "Action (%)"() -> (w4638:dbl)
                                n2846 = Absolute Value(x=w4638) -> (abs(x)=w4637:dbl)
                                n2847 = Greater?(x=w4637, y=70.0) -> (0:w4635:bool)
                                n2848 = property on="Remove Action Offset" class="Bool (strict)"("Val(Sgnl)"=w4635) -> ()  [unwired: 2 in, 2 out]
                                }
                                frame #3 {
                                n2849 = for {
                                N: 4 -> [_]
                                n2850 = flat-sequence {
                                frame #0 {
                                n2851 = Wait (ms)(milliseconds to wait=u32 500) -> ()  [unwired: 1 out]
                                }
                                frame #1 {
                                n2852 = local read "Action (%)"() -> (w4644:dbl)
                                n2853 = Absolute Value(x=w4644) -> (abs(x)=w4643:dbl)
                                n2854 = Greater?(x=w4643, y=70.0) -> (0:w4641:bool)
                                n2855 = property on="Remove Action Offset" class="Bool (strict)"("Val(Sgnl)"=w4641) -> ()  [unwired: 2 in, 2 out]
                                }
                                }
                                }
                                }
                                frame #4 {
                                n2856 = Wait (ms)(milliseconds to wait=u32 500) -> ()  [unwired: 1 out]
                                }
                                frame #5 {
                                n2857 = local read "Shift confocal"() -> (w4649:bool)
                                n2858 = local read "Mean"() -> (w4652:dbl)
                                n2859 = Greater?(x=w4652, y=11.0) -> (0:w4648:bool)
                                n2860 = Not(x=w4648) -> (.not. x?=w4647:bool)
                                n2861 = And(x=w4648, y=w4649) -> (x .and. y?=w4650:bool)
                                n2862 = And(x=w4647, y=w4649) -> (x .and. y?=w4646:bool)
                                n2863 = case shown="True" w4650 {
                                frame False {
                                }
                                frame True {
                                n2864 = local read "Confocal X 2 (V)"() -> (w4655:dbl)
                                n2865 = local read "Confocal Y 2 (V)"() -> (w4656:dbl)
                                n2866 = property on="AO2" class="Slide (strict)"("Val(Sgnl)"=w4655) -> ()  [unwired: 2 in, 2 out]
                                n2867 = property on="AO1" class="Slide (strict)"("Val(Sgnl)"=w4656) -> ()  [unwired: 2 in, 2 out]
                                }
                                }
                                n2868 = case shown="True" w4646 {
                                frame False {
                                }
                                frame True {
                                n2869 = local read "Confocal Y 1 (V)"() -> (w4654:dbl)
                                n2870 = local read "Confocal X 1 (V)"() -> (w4653:dbl)
                                n2871 = property on="AO1" class="Slide (strict)"("Val(Sgnl)"=w4654) -> ()  [unwired: 2 in, 2 out]
                                n2872 = property on="AO2" class="Slide (strict)"("Val(Sgnl)"=w4653) -> ()  [unwired: 2 in, 2 out]
                                }
                                }
                                }
                                frame #6 {
                                n2873 = Wait (ms)(milliseconds to wait=u32 1500) -> ()  [unwired: 1 out]
                                }
                                frame #7 {
                                n2874 = property on="Rem fb disp offset" class="Bool (strict)"("Val(Sgnl)"=TRUE ("Value (Signaling)")) -> ()  [unwired: 2 in, 2 out]
                                }
                                }
                                }
                                frame True {
                                n2875 = flat-sequence {
                                tunnel: w4659 -> [w4660]
                                frame #0 {
                                n2876 = property on="Trap Delta (MHz)" class="DigNum (strict)"("Val(Sgnl)"=w4660) -> ()  [unwired: 2 in, 2 out]
                                }
                                frame #1 {
                                n2877 = Wait (ms)(milliseconds to wait=u32 500) -> ()  [unwired: 1 out]
                                }
                                frame #2 {
                                n2878 = local read "Shift confocal"() -> (w4666:bool)
                                n2879 = local read "Mean"() -> (w4667:dbl)
                                n2880 = Greater?(x=w4667, y=11.0) -> (0:w4665:bool)
                                n2881 = And(x=w4665, y=w4666) -> (x .and. y?=w4663:bool)
                                n2882 = Not(x=w4665) -> (.not. x?=w4664:bool)
                                n2883 = And(x=w4664, y=w4666) -> (x .and. y?=w4662:bool)
                                n2884 = case shown="True" w4663 {
                                frame False {
